vi "Load Music.vi"(8 "error in (no error)":errorcluster, 10 "Supported Music Libraries Paths":path[](array[path])=[path "C:/Users/devonf/Desktop/Reno/Test/BAMP3/plugins/Supported Music Libraries/SPX/SPXMusicLibrary.lvclass"], 11 "Music Folder":path=path "C:/Users/devonf/Desktop/Reno/Test/Instructions") -> (0 "error out":errorcluster, 3 "MusicLibrary":refnum<class "MusicLibrary.lvclass">)   [LabVIEW 2015, in "MusicFile.lvclass"]
uses:
  MusicFile.lvclass
  MusicElementLibrary/MusicLibrary/MusicLibrary.lvclass
  MusicFile.lvclass/MusicFile.ctl
  MusicElementLibrary/MusicElementLibrary.lvclass
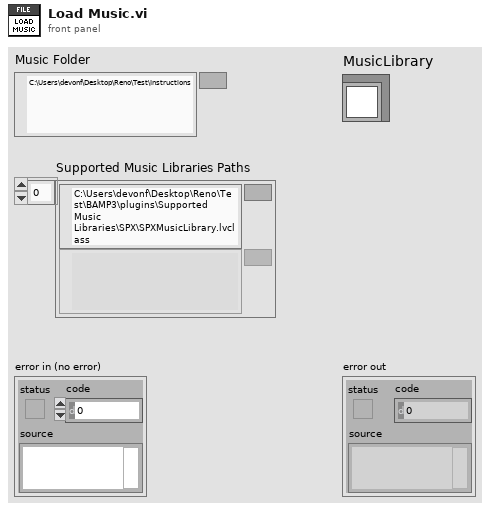
[diagram p1: front panel]
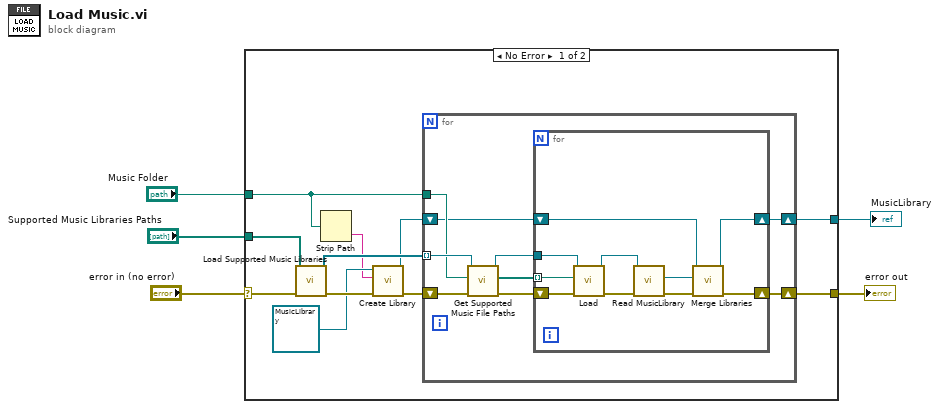
[diagram p0: block diagram]
diagram:
  n1 = case shown="No Error" "error in (no error)" {
    selector: "error in (no error)" -> [w16 w36]
    tunnel: [w13 w36] -> w4
    tunnel: "Supported Music Libraries Paths" -> [w15 _]
    tunnel: "Music Folder" -> [w8 _]
    tunnel: [w6 _] -> w1
    frame No Error {
      n2 = call "Load Supported Music Libraries.vi"("error in (no error)"=w16, "Supported Music Libraries Paths"=w15) -> ("error out"=w12:errorcluster, "Supported Files"=w14:refnum<class "MusicFile.lvclass">[])  [unwired: 8 in]
      n3 = Strip Path(path=w8) -> (name=w7:string)  [unwired: 1 out]
      n4 = call "Create Library.vi"("error in (no error)"=w12, "Name"=w7, "MusicElementLibrary in"=refnum<class "MusicLibrary.lvclass"> refnum ("MusicLibrary.lvclass")) -> ("error out"=w11:errorcluster, "MusicElementLibrary out"=w9:refnum<class "MusicLibrary.lvclass">)  [unwired: 7 in]
      n5 = for {
        tunnel: w14 -> [w22] mode=indexing
        tunnel: w8 -> [w21]
        shift-right: [w25] -> w13
        shift-left: w11 -> [w24]
        shift-right: [w17] -> w6
        shift-left: w9 -> [w18]
        n6 = call "Get Supported Music File Paths.vi"("error in (no error)"=w24, "Music Folder Path"=w21, "MusicFile In"=w22) -> ("error out"=w23:errorcluster, "Music File Paths"=w19:path[], "MusicFile Out"=w20:refnum<class "MusicFile.lvclass">)  [unwired: 6 in]
        n7 = for {
          tunnel: w20 -> [w34]
          shift-right: [w29] -> w25
          shift-left: w23 -> [w35]
          tunnel: w19 -> [w33] mode=indexing
          shift-right: [w26] -> w17
          shift-left: w18 -> [w28]
          n8 = call-dynamic "Load.vi"("error in (no error)"=w35, "File"=w33, "MusicFile In"=w34) -> ("error out"=w32:errorcluster, "MusicFile Out"=w31:refnum<class "MusicFile.lvclass">)  [unwired: 7 in]
          n9 = call "Read MusicLibrary.vi"("error in (no error)"=w32, "MusicFile in"=w31) -> ("error out"=w30:errorcluster, "MusicLibrary.lvclass"=w27:refnum<class "MusicLibrary.lvclass">)  [unwired: 7 in, 1 out]
          n10 = call "Merge Libraries.vi"("error in (no error)"=w30, "MusicLibrary To Merge"=w27, "MusicLibrary in"=w28) -> ("error out"=w29:errorcluster, "MusicLibrary out"=w26:refnum<class "MusicLibrary.lvclass">)  [unwired: 7 in]
        }
      }
    }
    frame Error {
    }
  }
  "error out" <- w4
  "MusicLibrary" <- w1
